vi "Jednoręki Bandyta 2.vi"() -> ()   [LabVIEW 2020]
panel:
  in  "OK Button":bool
  out "Wynik!":string
  out "3":dbl
  in  "stop 3":bool
  out "2":dbl
  in  "stop 2":bool
  out "1":dbl
  in  "stop":bool
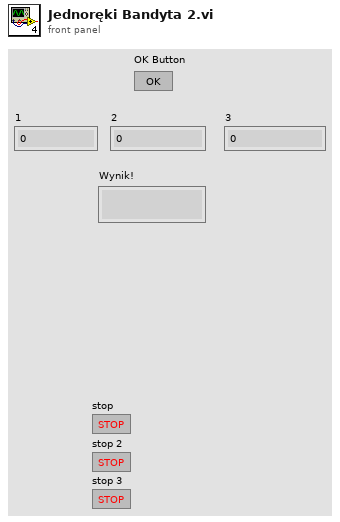
[diagram p1: front panel]
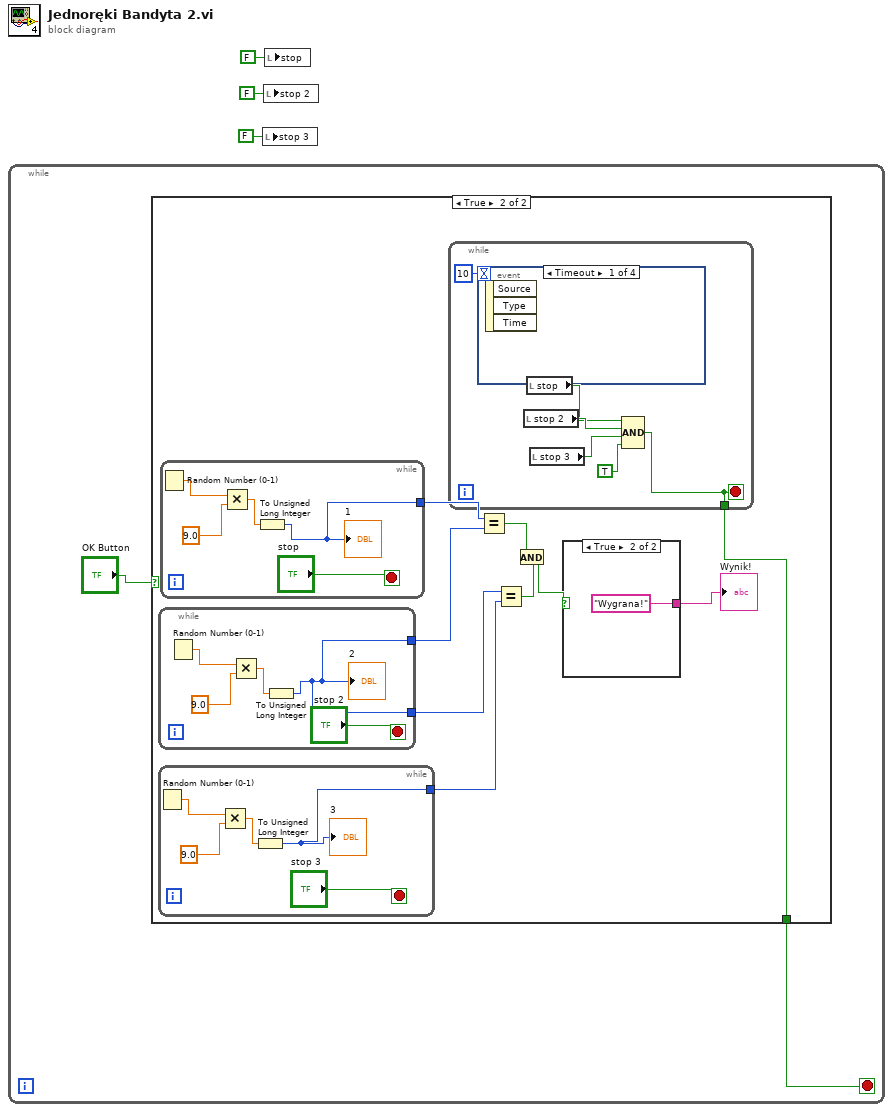
[diagram p0: block diagram]
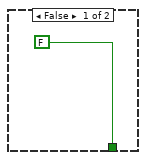
[diagram p2: hidden frame]
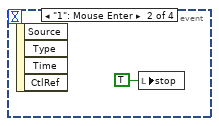
[diagram p3: hidden frame]
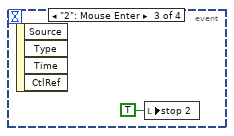
[diagram p4: hidden frame]
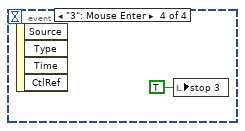
[diagram p5: hidden frame]
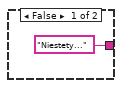
[diagram p6: hidden frame]
diagram:
  n1 = while {
    stop <- w4 stop-if-true
    n2 = case shown="True" "OK Button" {
      tunnel: [FALSE w7] -> w4
      frame False {
      }
      frame True {
        n3 = while {
          tunnel: [w33] -> w14
          tunnel: [w33] -> w13
          stop <- "stop 2" stop-if-true
          n4 = Random Number (0-1)() -> (number: 0 to 1=w36:dbl)
          n5 = Multiply(x=w36, y=9.0) -> (x*y=w35:dbl)
          n6 = To Unsigned Long Integer(number=w35) -> (unsigned 32bit integer=w33:u32)
          "2" <- w33
        }
        n7 = while {
          tunnel: [w28] -> w12
          stop <- "stop 3" stop-if-true
          n8 = Random Number (0-1)() -> (number: 0 to 1=w30:dbl)
          n9 = Multiply(x=w30, y=9.0) -> (x*y=w31:dbl)
          n10 = To Unsigned Long Integer(number=w31) -> (unsigned 32bit integer=w28:u32)
          "3" <- w28
        }
        n11 = while {
          tunnel: [w38] -> w15
          stop <- "stop" stop-if-true
          n12 = Random Number (0-1)() -> (number: 0 to 1=w40:dbl)
          n13 = Multiply(x=w40, y=9.0) -> (x*y=w41:dbl)
          n14 = To Unsigned Long Integer(number=w41) -> (unsigned 32bit integer=w38:u32)
          "1" <- w38
        }
        n15 = while {
          tunnel: [w17] -> w7
          stop <- w17 stop-if-true
          n16 = event shown="[0] Timeout" {
            selector: _ -> [_ _ _ _]
            dyn-events: _ -> [_ _ _ _]
            timeout: 10 -> [_ _ _ _]
            event Timeout {
              n17 = event-data() -> ()  [unwired: 1 in, 3 out]
            }
            event "1": Mouse Enter {
              n18 = event-data() -> ()  [unwired: 1 in, 4 out]
              n19 = local write "stop"(TRUE ("stop")) -> ()
            }
            event "2": Mouse Enter {
              n20 = event-data() -> ()  [unwired: 1 in, 4 out]
              n21 = local write "stop 2"(TRUE ("stop 2")) -> ()
            }
            event "3": Mouse Enter {
              n22 = event-data() -> ()  [unwired: 1 in, 4 out]
              n23 = local write "stop 3"(TRUE ("stop 3")) -> ()
            }
          }
          n24 = local read "stop 2"() -> (w20:bool)
          n25 = local read "stop"() -> (w19:bool)
          n26 = local read "stop 3"() -> (w21:bool)
          n27 = Compound Arithmetic op=AND(w19, w20, w21, TRUE ("value")) -> (w17:bool)
        }
        n28 = Equal?(x=w15, y=w14) -> (x = y?=w10:bool)
        n29 = Equal?(x=w13, y=w12) -> (x = y?=w9:bool)
        n30 = And(x=w10, y=w9) -> (x .and. y?=w11:bool)
        n31 = case shown="True" w11 {
          tunnel: ["Niestety..." ("String") "Wygrana!"] -> w8
          frame False {
          }
          frame True {
          }
        }
        "Wynik!" <- w8
      }
    }
  }
  n32 = local write "stop 3"(FALSE ("stop 3")) -> ()
  n33 = local write "stop 2"(FALSE ("stop 2")) -> ()
  n34 = local write "stop"(FALSE ("stop")) -> ()
